vi "Filter Partnumbers.vi"(10 "Array in":refnum<class "Symbol.lvclass">[](array[class]), 11 "Array 3":refnum<class "Number.lvclass">[](array[class])) -> (3 "Array out":refnum<class "Number.lvclass">[](array[class]))   [LabVIEW 2020, in "Schema Parser.lvclass"]
uses:
  Schema Parser.lvclass
  Number/Number.lvclass
  Symbol/Symbol.lvclass
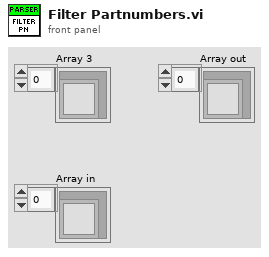
[diagram p1: front panel]
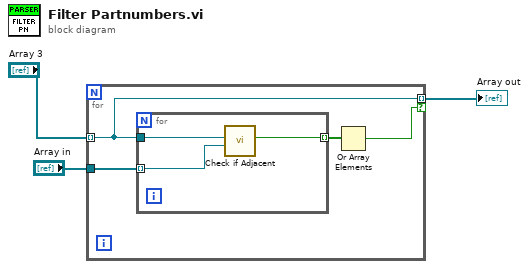
[diagram p0: block diagram]
diagram:
  n1 = for {
    tunnel: "Array 3" -> [w5] mode=indexing
    tunnel: "Array in" -> [w7]
    tunnel: [w5] -> w3 mode=indexing if=w4
    n2 = for {
      tunnel: w5 -> [w10]
      tunnel: w7 -> [w9] mode=indexing
      tunnel: [w8] -> w6 mode=indexing
      n3 = call "Check if Adjacent.vi"("Symbol.lvclass"=w9, "Number.lvclass"=w10) -> ("Is Adjacent?"=w8:bool)  [unwired: 8 in, 1 out]
    }
    n4 = Or Array Elements(Boolean array=w6) -> (logical OR=w4:bool)
  }
  "Array out" <- w3
